vi "Corr Digitizer Load INFO.vi"(7 "item ref":refnum<vi>, 8 "error in":errorcluster, 11 "Path":path) -> (0 "error out":errorcluster, 3 "digitizer info":T1)   [LabVIEW 2013]
doc: "Loads digitizer INFO file."
uses:
  Corr Digitizer INFO.ctl
  Corr Digitizer INFO item.ctl
  Corr Digitizer INFO parameter.ctl
  octave/infolib.lvlibp/Private/Get key polymorph parts/GetString.vi
  octave/infolib.lvlibp/Private/Get matrix polymorph parts/Get 1D String.vi
  <vilib>/Utility/error.llb/Error Cluster From Error Code.vi
  octave/infolib.lvlibp/Private/Get matrix polymorph parts/Get 2D String.vi
  octave/infolib.lvlibp/Private/Get key polymorph parts/GetI64.vi
  <vilib>/ErrorRing/Error Ring.xnode
  octave/infolib.lvlibp
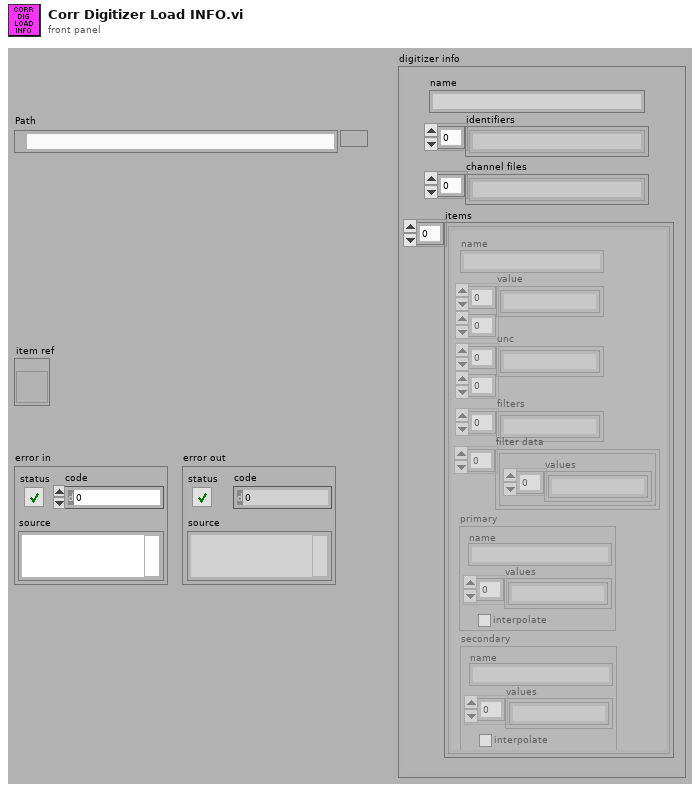
[diagram p1: front panel]
types:
  T1 = typedef "Corr Digitizer INFO.ctl" = cluster{"name":string, "identifiers":string[], "channel files":string[], "items":T2[]}
  T2 = typedef "Corr Digitizer INFO item.ctl" = cluster{"name":string, "value":string[][], "unc":string[][], "filters":string[], "primary":T3, "secondary":T3, "filter data":cluster{"values":string[]}[]}
  T3 = typedef "Corr Digitizer INFO parameter.ctl" = cluster{"values":string[], "interpolate":bool, "name":string}
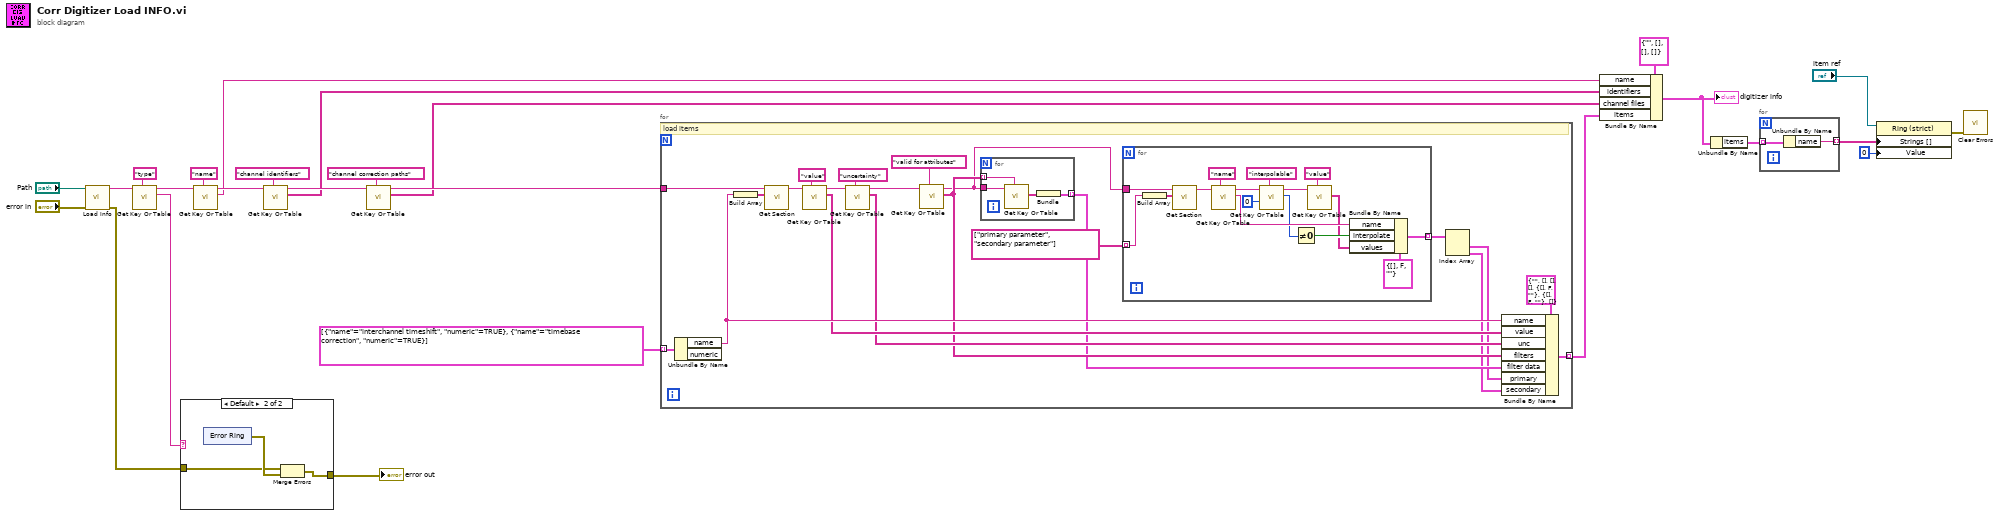
[diagram p0: block diagram]
diagram:
  n1 = call "Load Info.vi"("error in"="error in", "filename"="Path") -> ("error out"=w8:errorcluster, "info data"=w24:string)  [unwired: 8 in]
  n2 = call-poly "Get Key Or Table.vi"("key description"="type", "info data"=w24) -> ("value"=w9:string, "info data out"=w22:string)  [unwired: 6 in, 2 out]
  n3 = case shown="Default" w9 {
    tunnel: w8 -> [w27 w29]
    tunnel: [w27 w28] -> w7
    frame "divider", "shunt" {
    }
    frame Default {
      n4 = xnode "Error Ring"() -> ("error out"=w30:errorcluster)
      n5 = Merge Errors(w29, w30) -> (w28:errorcluster)
    }
  }
  "error out" <- w7
  n6 = call-poly "Get Key Or Table.vi"("key description"="name", "info data"=w22) -> ("value"=w5:string, "info data out"=w14:string)  [unwired: 6 in, 2 out]
  n7 = call-poly "Get Key Or Table.vi"("key description"="channel identifiers", "info data"=w14) -> ("value"=w4:string[], "info data out"=w11:string)  [unwired: 6 in, 2 out]
  n8 = call-poly "Get Key Or Table.vi"("key description"="channel correction paths", "info data"=w11) -> ("value"=w3:string[], "info data out"=w10:string)  [unwired: 6 in, 2 out]
  n9 = for {
    tunnel: cluster{"name":string, "numeric":bool}[] [{"name"="interchannel timeshift", "numeric"=TRUE}, {"name"="timebase correction", "numeric"=TRUE}] -> [w56] mode=indexing
    tunnel: w10 -> [w54]
    tunnel: [w55] -> w1 mode=indexing
    # "load items"
    n10 = Unbundle By Name(w56) -> ("name"=w49:string)  [unwired: 1 out]
    n11 = Build Array(w49) -> (w53:string[])
    n12 = call "Get Section.vi"("sections"=w53, "info data"=w54) -> ("section part"=w52:string)  [unwired: 8 in, 1 out]
    n13 = call-poly "Get Key Or Table.vi"("key description"="value", "info data"=w52) -> ("value"=w47:string[][], "info data out"=w46:string)  [unwired: 6 in, 2 out]
    n14 = call-poly "Get Key Or Table.vi"("key description"="uncertainty", "info data"=w46) -> ("value"=w45:string[][], "info data out"=w43:string)  [unwired: 6 in, 2 out]
    n15 = call-poly "Get Key Or Table.vi"("key description"="valid for attributes", "info data"=w43) -> ("value"=w42:string[], "info data out"=w40:string)  [unwired: 6 in, 2 out]
    n16 = for {
      tunnel: w40 -> [w76]
      tunnel: w42 -> [w75] mode=indexing
      tunnel: [w73] -> w41 mode=indexing
      n17 = call-poly "Get Key Or Table.vi"("key description"=w75, "info data"=w76) -> ("value"=w74:string[])  [unwired: 6 in, 3 out]
      n18 = Bundle("value"=w74) -> (w73:cluster{"value":string[]})  [unwired: 1 in]
    }
    n19 = for {
      tunnel: w40 -> [w72]
      tunnel: string[] ["primary parameter", "secondary parameter"] -> [w71] mode=indexing
      tunnel: [w58] -> w38 mode=indexing
      n20 = Build Array(w71) -> (w70:string[])
      n21 = call "Get Section.vi"("sections"=w70, "info data"=w72) -> ("section part"=w68:string)  [unwired: 8 in, 1 out]
      n22 = call-poly "Get Key Or Table.vi"("key description"="name", "info data"=w68) -> ("value"=w66:string, "info data out"=w64:string)  [unwired: 6 in, 2 out]
      n23 = call-poly "Get Key Or Table.vi"("key description"="interpolable", "numeric"=i64 0, "info data"=w64) -> ("value"=w63:i64, "info data out"=w62:string)  [unwired: 5 in, 2 out]
      n24 = Not Equal To 0?(x=w63) -> (x != 0?=w61:bool)
      n25 = call-poly "Get Key Or Table.vi"("key description"="value", "info data"=w62) -> ("value"=w59:string[])  [unwired: 6 in, 3 out]
      n26 = Bundle By Name(cluster=T3 {"values"=[], "interpolate"=FALSE, "name"=""} ("primary data"), "name"=w66, "interpolate"=w61, "values"=w59) -> (w58:T3)
    }
    n27 = Index Array(array=w38) -> (element #1=w37:T3, element #2=w36:T3)  [unwired: 2 in]
    n28 = Bundle By Name(cluster=T2 {"name"="", "value"=[], "unc"=[], "filters"=[], "primary"={"values"=[], "interpolate"=FALSE, "name"=""}, "secondary"={"values"=[], "interpolate"=FALSE, "name"=""}, "filter data"=[]} ("correction"), "name"=w49, "value"=w47, "unc"=w45, "filters"=w42, "filter data"=w41, "primary"=w37, "secondary"=w36) -> (w55:T2)
  }
  n29 = Bundle By Name(cluster=T1 {"name"="", "identifiers"=[], "channel files"=[], "items"=[]} ("digitizer info"), "name"=w5, "identifiers"=w4, "channel files"=w3, "items"=w1) -> (w2:T1)
  "digitizer info" <- w2
  n30 = Unbundle By Name(w2) -> ("items"=w21:T2[])
  n31 = for {
    tunnel: w21 -> [w78] mode=indexing
    tunnel: [w77] -> w19 mode=indexing
    n32 = Unbundle By Name(w78) -> ("name"=w77:string)
  }
  n33 = property class="Ring (strict)"(reference="item ref", "Strings []"=w19, "Value"=u16 0) -> (error out=w17:errorcluster)  [unwired: 1 in, 1 out]
  n34 = call <vilib>:"Clear Errors.vi"("error in (no error)"=w17) -> ()  [unwired: 6 in, 1 out]
